vi "transfer_and_submit_job.vi"(6 "Mapped Remote Directory Path":string, 7 "Date Folder":string, 8 "Password":string, 9 "Username":string, 10 "Remote Data Directory":string, 11 "Local Data Directory":string) -> ()   [LabVIEW 2014]
panel:
  out "standard error":string
  out "standard output":string
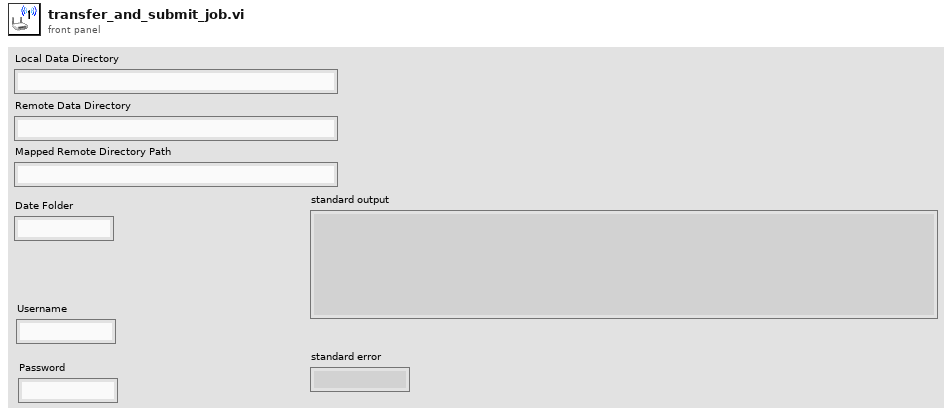
[diagram p1: front panel]
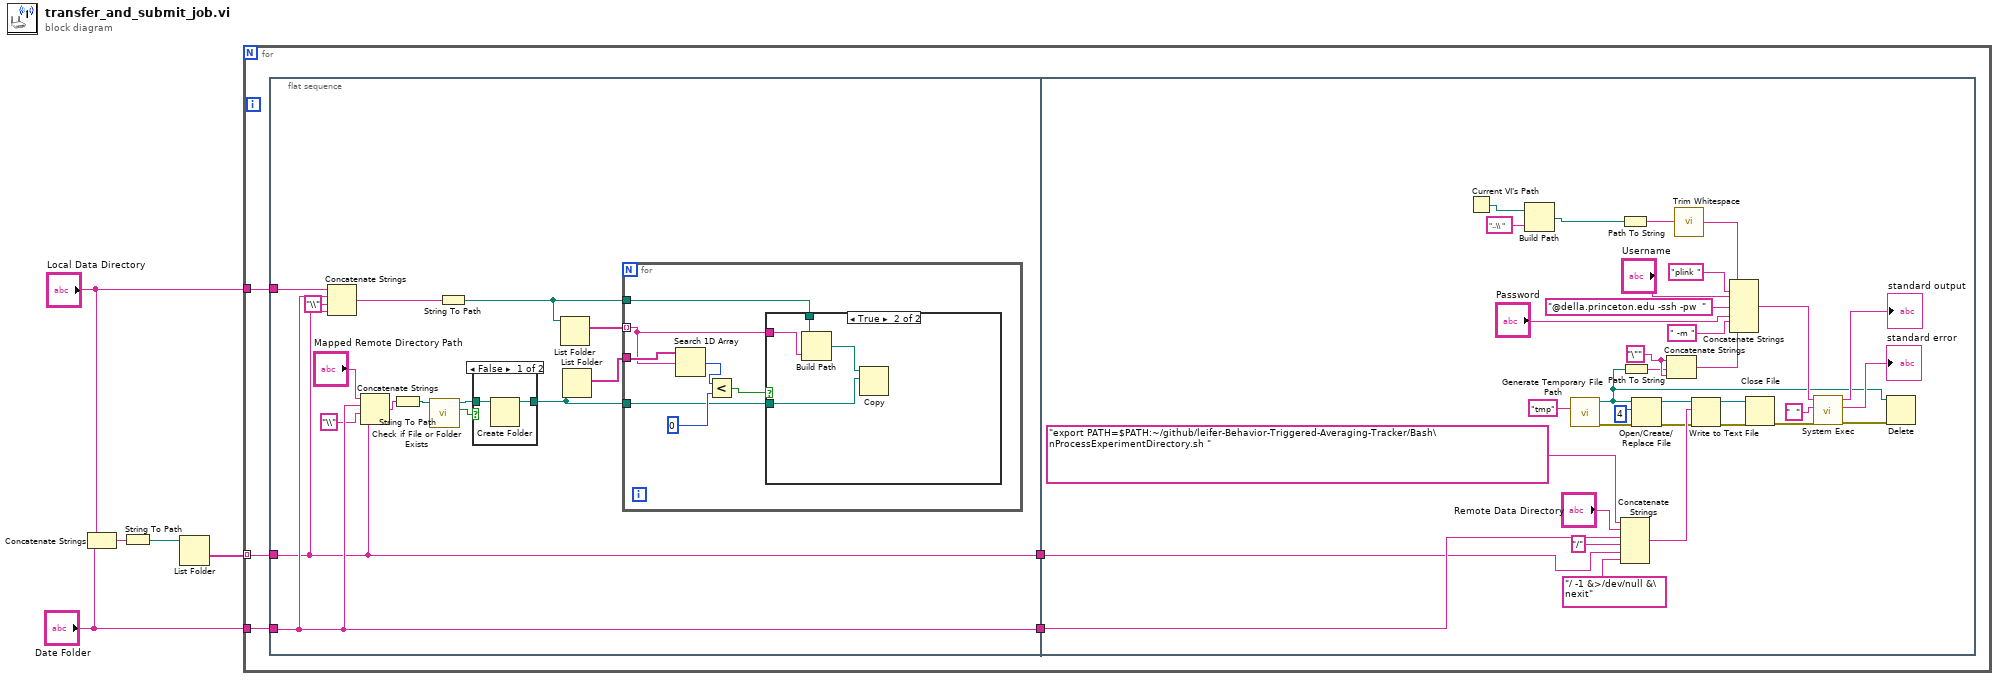
[diagram p0: block diagram]
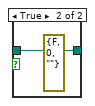
[diagram p2: hidden frame]
diagram:
  n1 = Concatenate Strings("Local Data Directory", "Date Folder") -> (w3:string)
  n2 = String To Path(string=w3) -> (path=w2:path)
  n3 = List Folder(path=w2) -> (folder names=w1:string[])  [unwired: 3 in, 3 out]
  n4 = for {
    tunnel: "Date Folder" -> [w8]
    tunnel: "Local Data Directory" -> [w7]
    tunnel: w1 -> [w6] mode=indexing
    n5 = flat-sequence {
      tunnel: [w18] -> w9
      tunnel: w8 -> [w18]
      tunnel: w6 -> [w15]
      tunnel: [w15] -> w10
      tunnel: w7 -> [w12]
      tunnel: w10 -> [w41]
      tunnel: w9 -> [w42]
      frame #0 {
        n6 = Concatenate Strings(w12, w18, "\\", w15) -> (w13:string)
        n7 = Concatenate Strings("Mapped Remote Directory Path", w18, "\\", w15) -> (w17:string)
        n8 = String To Path(string=w17) -> (path=w20:path)
        n9 = call <vilib>:"Check if File or Folder Exists.vi"("path"=w20) -> ("file or folder exists?"=w22:bool, "dup path"=w21:path)  [unwired: 8 in, 1 out]
        n10 = String To Path(string=w13) -> (path=w14:path)
        n11 = case shown="False" w22 {
          tunnel: [w26 w28] -> w19
          tunnel: w21 -> [w27 w28]
          frame False {
            n12 = Create Folder(path (use dialog)=w27) -> (created path=w26:path)  [unwired: 2 in, 2 out]
          }
          frame True {
            (unwired) errorcluster {"status"=FALSE, "code"=0, "source"=""} ("error out")
          }
        }
        n13 = List Folder(path=w14) -> (filenames=w25:string[])  [unwired: 3 in, 3 out]
        n14 = List Folder(path=w19) -> (filenames=w24:string[])  [unwired: 3 in, 3 out]
        n15 = for {
          tunnel: w25 -> [w30] mode=indexing
          tunnel: w24 -> [w32]
          tunnel: w19 -> [w31]
          tunnel: w14 -> [w29]
          n16 = Search 1D Array(1D array=w32, element=w30) -> (index of element=w35:i32)  [unwired: 1 in]
          n17 = Less?(x=w35, y=0) -> (x < y?=w33:bool)
          n18 = case shown="True" w33 {
            tunnel: w30 -> [_ w38]
            tunnel: w31 -> [_ w39]
            tunnel: w29 -> [_ w37]
            frame False {
            }
            frame True {
              n19 = Build Path(base path=w37, name or relative path=w38) -> (appended path=w36:path)
              n20 = Copy(10:w39, 11:w36) -> ()  [unwired: 3 in, 3 out]
            }
          }
        }
      }
      frame #1 {
        w63 = "\""
        n21 = Current VI's Path() -> (path=w68:path)
        n22 = Build Path(base path=w68, name or relative path="..\\ ") -> (appended path=w70:path)
        n23 = call <vilib>:"Generate Temporary File Path.vi"("Temporary File Extension (tmp)"="tmp") -> ("error out"=w45:errorcluster, "Unique Temporary File Path"=w51:path)  [unwired: 9 in]
        n24 = Path To String(path=w70) -> (string=w71:string)
        n25 = Concatenate Strings("export PATH=$PATH:~/github/leifer-Behavior-Triggered-Averaging-Tracker/Bash\nProcessExperimentDirectory.sh ", "Remote Data Directory", w42, "/", w41, "/ -1 &>/dev/null &\nexit") -> (w53:string)
        n26 = Path To String(path=w51) -> (string=w61:string)
        n27 = Open/Create/Replace File(file path (use dialog)=w51, error in=w45, operation (0:open)=4) -> (refnum out=w46:refnum<file>, error out=w43:errorcluster)  [unwired: 3 in, 1 out]
        n28 = Concatenate Strings(w63, w61, w63) -> (w62:string)
        n29 = call <vilib>:"Trim Whitespace.vi"("string"=w71) -> ("trimmed string"=w72:string)  [unwired: 1 in]
        n30 = Write to Text File(file (use dialog)=w46, text=w53, error in=w43) -> (refnum out=w47:refnum<file>, error out=w44:errorcluster)  [unwired: 1 in, 1 out]
        n31 = Concatenate Strings(w72, "plink ", "Username", "@della.princeton.edu -ssh -pw  ", "Password", " -m ", w62) -> (w64:string)
        n32 = Close File(refnum=w47, error in=w44) -> (error out=w48:errorcluster)  [unwired: 1 out]
        n33 = call <vilib>:"System Exec.vi"("error in (no error)"=w48, "standard input"="  ", "command line"=w64) -> ("error out"=w49:errorcluster, "standard error"=→"standard error":string, "standard output"=→"standard output":string)  [unwired: 5 in, 1 out]
        n34 = Delete(path (use dialog)=w51, error in=w49) -> ()  [unwired: 3 in, 3 out]
      }
    }
  }
